vi "Reorder Frames.vi"(7 "Num Event Frames":i32, 8 "error in (no error)":errorcluster, 9 "Desired Frame Ordering":string[](array[string]), 10 "Original Frame Ordering":string[](array[string]), 11 "JKI SM in":refnum<class "JKI SM.lvclass">) -> (0 "error out":errorcluster)   [LabVIEW 2013]
uses:
  JKI State Machine API/source/JKI SM/JKI SM.lvclass
  JKI State Machine API/source/JKI SM/JKI SM.lvclass/JKI SM.ctl
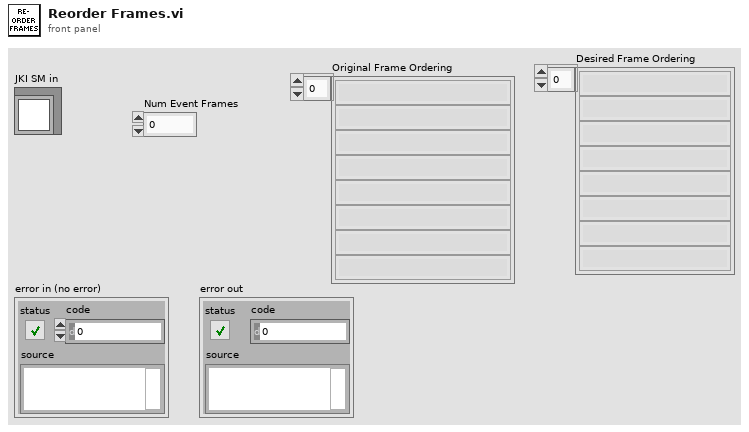
[diagram p1: front panel]
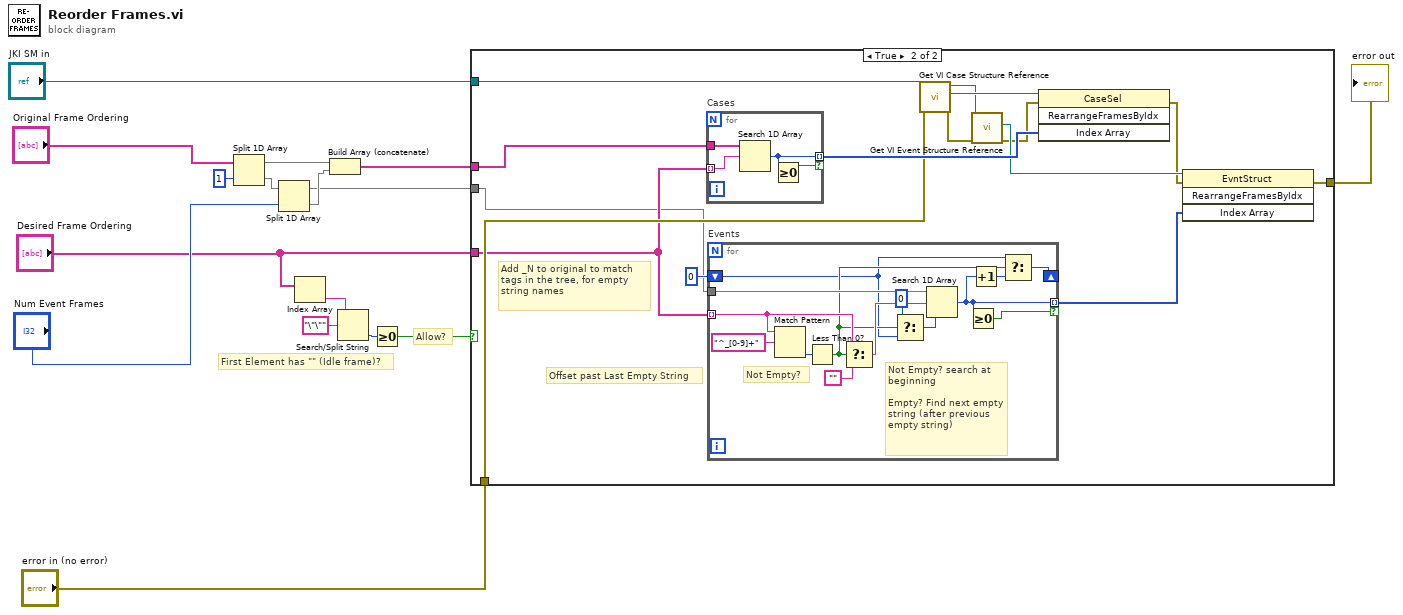
[diagram p0: block diagram]
diagram:
  # "Allow?"
  # "First Element has \"\" (Idle frame)?"
  n1 = Split 1D Array(array="Original Frame Ordering", index=1) -> (first subarray=w14:string[], second subarray=w12:string[])
  n2 = Split 1D Array(array=w12, index="Num Event Frames") -> (first subarray=w9:string[], second subarray=w11:string[])
  n3 = Index Array(array="Desired Frame Ordering") -> (element=w3:string)  [unwired: 1 in]
  n4 = Build Array (concatenate)(w14, w11) -> (w10:string[])
  n5 = Search/Split String(string=w3, search string/char (-)="\"\"") -> (offset of match=w2:i32)  [unwired: 1 in, 2 out]
  n6 = Greater Or Equal To 0?(x=w2) -> (x >= 0?=w1:bool)
  n7 = case shown="True" w1 {
    tunnel: w10 -> [_ w31]
    tunnel: w9 -> [_ w18]
    tunnel: "JKI SM in" -> [_ w30]
    tunnel: "error in (no error)" -> [w17 w28]
    tunnel: [w17 w22] -> w6
    tunnel: "Desired Frame Ordering" -> [_ w21]
    frame False {
    }
    frame True {
      # "Offset past Last Empty String"
      # "Add _N to original to match tags in the tree, for empty string names"
      n8 = for "Cases" {
        tunnel: w31 -> [w50]
        tunnel: w21 -> [w49] mode=indexing
        tunnel: [w48] -> w32 mode=indexing if=w47
        n9 = Search 1D Array(1D array=w50, element=w49) -> (index of element=w48:i32)  [unwired: 1 out]
        n10 = Greater Or Equal To 0?(x=w48) -> (x >= 0?=w47:bool)
      }
      n11 = for "Events" {
        tunnel: w18 -> [w46]
        tunnel: w21 -> [w38] mode=indexing
        tunnel: [w41] -> w19 mode=indexing if=w45
        shift-right: [w40] -> _
        shift-left: 0 ("start index (0)") -> [w35]
        # "Not Empty? search at beginning\n\nEmpty? Find next empty string (after previous empty string)"
        # "Not Empty?"
        n12 = Match Pattern(string=w38, regular expression="^_[0-9]+") -> (offset past match=w43:i32)  [unwired: 1 in, 3 out]
        n13 = Less Than 0?(x=w43) -> (x < 0?=w36:bool)
        n14 = Select(t=w38, s=w36, f="") -> (s? t:f=w37:string)
        n15 = Select(t=0, s=w36, f=w35) -> (s? t:f=w34:i32)
        n16 = Search 1D Array(1D array=w46, element=w37, start index (0)=w34) -> (index of element=w41:i32)
        n17 = Greater Or Equal To 0?(x=w41) -> (x >= 0?=w45:bool)
        n18 = Increment(x=w41) -> (x+1=w39:i32)
        n19 = Select(t=w35, s=w36, f=w39) -> (s? t:f=w40:i32)
      }
      n20 = call "Get VI Case Structure Reference.vi"("error in (no error)"=w28, "JKI SM in"=w30) -> ("error out"=w26:errorcluster, "Case Structure ref"=w29:refnum<vi>, "JKI SM out"=w27:refnum<class "JKI SM.lvclass">)  [unwired: 7 in]
      n21 = call "Get VI Event Structure Reference.vi"("error in (no error)"=w26, "JKI SM in"=w27) -> ("error out"=w24:errorcluster, "Event Structure ref"=w25:refnum<vi>)  [unwired: 7 in, 1 out]
      n22 = invoke class="CaseSel" method="RearrangeFramesByIdx"(reference=w29, error in=w24, "Index Array"=w32) -> (error out=w23:errorcluster)  [unwired: 1 in, 3 out]
      n23 = invoke class="EvntStruct" method="RearrangeFramesByIdx"(reference=w25, error in=w23, "Index Array"=w19) -> (error out=w22:errorcluster)  [unwired: 1 in, 3 out]
    }
  }
  "error out" <- w6
